vi "PC_CallRTFireAndForget.vi"(4 "Value":variant, 6 "Control Name":string="InputControl", 7 "Machine":string="192.168.120.8", 8 "error in (no error)":errorcluster, 9 "SetControl?":bool, 10 "Reentrant?":bool, 11 "VIPath":path=path "C:/ni-rt/startup/Test.vi") -> (0 "error out":errorcluster, 3 "reference out":refnum<vi>)   [LabVIEW 2010]
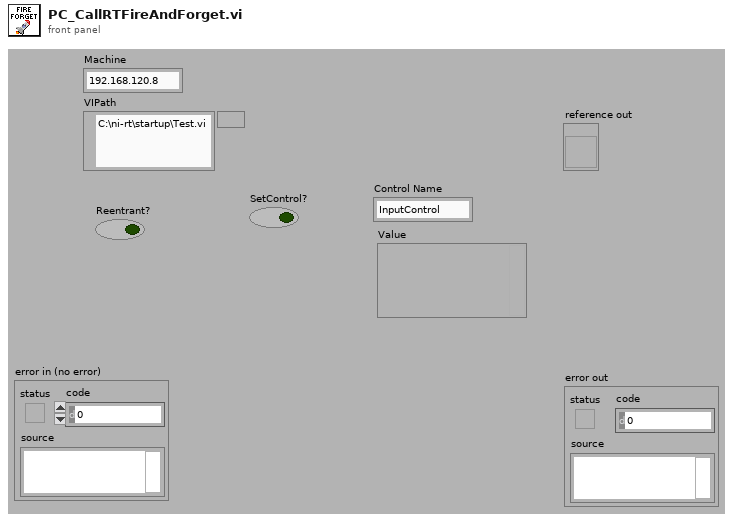
[diagram p1: front panel]
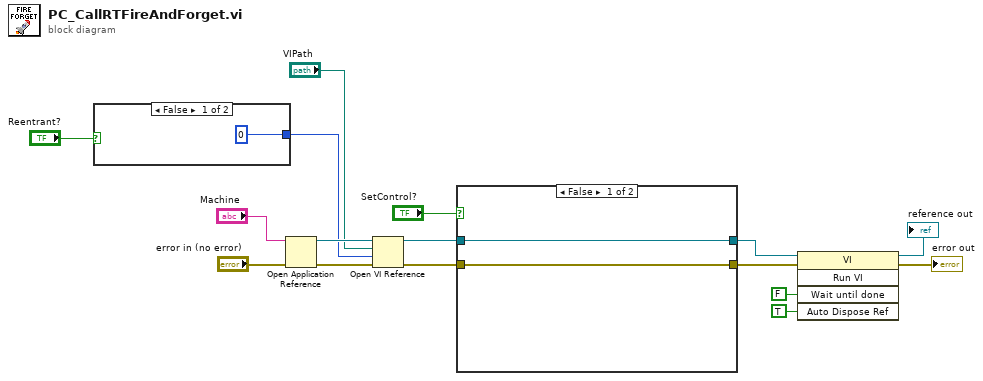
[diagram p0: block diagram]
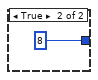
[diagram p2: hidden frame]
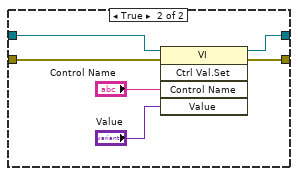
[diagram p3: hidden frame]
diagram:
  n1 = case shown="False" "Reentrant?" {
    tunnel: [0 ("options") 8 ("options")] -> w10
    frame False {
    }
    frame True {
    }
  }
  n2 = Open Application Reference(8:"error in (no error)", 11:"Machine") -> (0:w14:errorcluster, 3:w15:refnum<vi>)  [unwired: 2 in]
  n3 = Open VI Reference(application reference (local)=w15, vi path="VIPath", options=w10, error in (no error)=w14) -> (vi reference=w9:refnum<vi>, error out=w7:errorcluster)  [unwired: 2 in]
  n4 = case shown="False" "SetControl?" {
    tunnel: w9 -> [w19 w25]
    tunnel: [w19 w24] -> w8
    tunnel: w7 -> [w20 w23]
    tunnel: [w20 w22] -> w6
    frame False {
    }
    frame True {
      n5 = invoke class="VI" method="Ctrl Val.Set"(reference=w25, error in=w23, "Control Name"="Control Name", "Value"="Value") -> (reference out=w24:refnum<vi>, error out=w22:errorcluster)  [unwired: 1 in, 3 out]
    }
  }
  n6 = invoke class="VI" method="Run VI"(reference=w8, error in=w6, "Wait until done"=FALSE ("Wait Until Done"), "Auto Dispose Ref"=TRUE ("Auto Dispose Reference")) -> (reference out=→"reference out":refnum<vi>, error out=→"error out":errorcluster)  [unwired: 1 in, 3 out]
